vi "SetVelocityArcade.vi"(9 "Y Axis":dbl, 10 "X Axis":dbl, 11 "DriveBase.lvclass":refnum<class "DriveBase.lvclass">) -> (3 "DriveBase.lvclass":refnum<class "DriveBase.lvclass">)   [LabVIEW 2016, in "DriveBase.lvclass"]
uses:
  DriveBase.lvclass
  DriveBase.lvclass/DriveBase.ctl
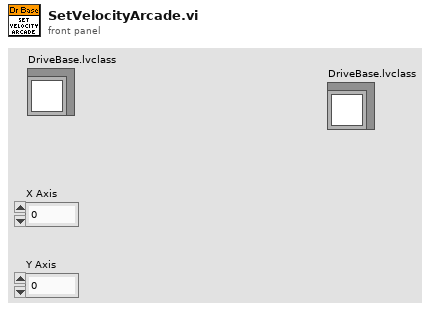
[diagram p1: front panel]
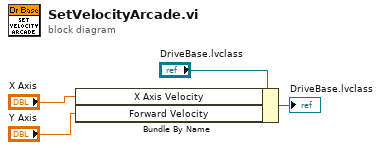
[diagram p0: block diagram]
diagram:
  n1 = Bundle By Name(cluster="DriveBase.lvclass", "X Axis Velocity"="X Axis", "Forward Velocity"="Y Axis") -> (→"DriveBase.lvclass":refnum<class "DriveBase.lvclass">)
